vi "NewPort_PM_AUTORANGE.vi"(8 "Error In":errorcluster, 9 "Stand Alone Mode":bool, 10 "USB Address":i32, 11 "reference":refnum<k24>) -> (0 "Error Out":errorcluster, 2 "Auto Range Enabled":bool, 3 "Query-String Format\nfrom Read Buffer":string)   [LabVIEW 2017]
uses:
  C:/Program Files (x86)/Newport/Newport USB Driver/Bin/UsbDllWrap.dll
  Program Files (x86)/Newport/Newport USB Driver/Bin/UsbDllWrap.dll
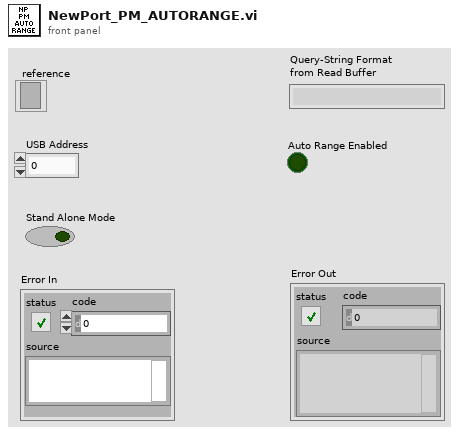
[diagram p1: front panel]
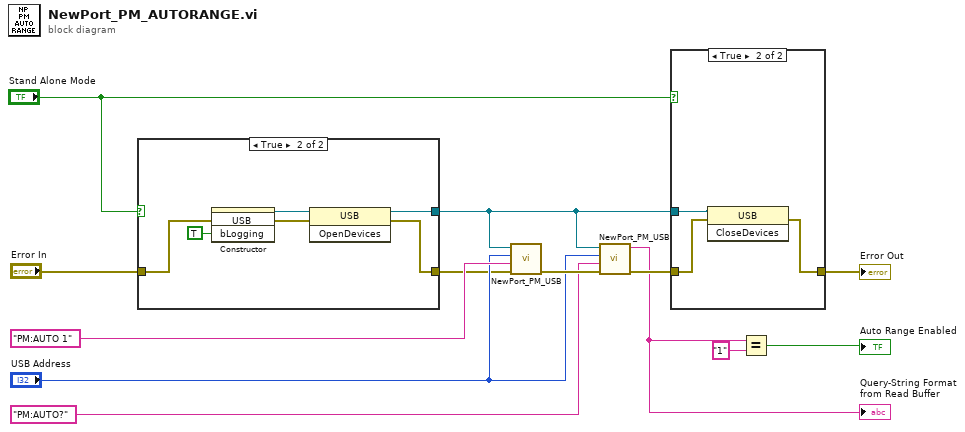
[diagram p0: block diagram]
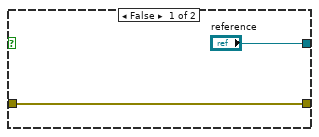
[diagram p3: hidden frame]
diagram:
  n1 = case shown="True" "Stand Alone Mode" {
    tunnel: ["reference" w21] -> w1
    tunnel: [w14 w20] -> w9
    tunnel: "Error In" -> [w14 w16]
    frame False {
    }
    frame True {
      n2 = constructor class="USB"(error in=w16, "bLogging"=TRUE) -> (reference out=w18:refnum<k24>, error out=w17:errorcluster)  [unwired: 2 in, 2 out]
      n3 = invoke class="USB" method="OpenDevices"(reference=w18, error in=w17) -> (reference out=w21:refnum<k24>, error out=w20:errorcluster)  [unwired: 1 in, 1 out]
    }
  }
  n4 = call "NewPort_PM_USB.vi"("error in"=w9, "PM:CMD_QUERY In"="PM:AUTO 1", "USB Address"="USB Address", "reference"=w1) -> ("error out"=w12:errorcluster)  [unwired: 5 in, 2 out]
  n5 = call "NewPort_PM_USB.vi"("error in"=w12, "PM:CMD_QUERY In"="PM:AUTO?", "USB Address"="USB Address", "reference"=w1) -> ("error out"=w6:errorcluster, "Query-String\nfrom Read Buffer\nComplete Info"=w4:string)  [unwired: 5 in, 1 out]
  "Query-String Format\nfrom Read Buffer" <- w4
  n6 = case shown="True" "Stand Alone Mode" {
    tunnel: w1 -> [_ w25]
    tunnel: w6 -> [w22 w24]
    tunnel: [w22 w23] -> w5
    frame False {
    }
    frame True {
      n7 = invoke class="USB" method="CloseDevices"(reference=w25, error in=w24) -> (error out=w23:errorcluster)  [unwired: 1 in, 2 out]
    }
  }
  "Error Out" <- w5
  n8 = Equal?(x=w4, y="1") -> (x = y?=→"Auto Range Enabled":bool)
